vi "Milan Box.vi"() -> ()   [LabVIEW 2019]
uses:
  <vilib>/httpClient/POSTBuffer.vi
  <vilib>/httpClient/LabVIEWHTTPClient.lvlib
panel:
  out "Property (time stamp)":timestamp
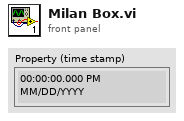
[diagram p1: front panel]
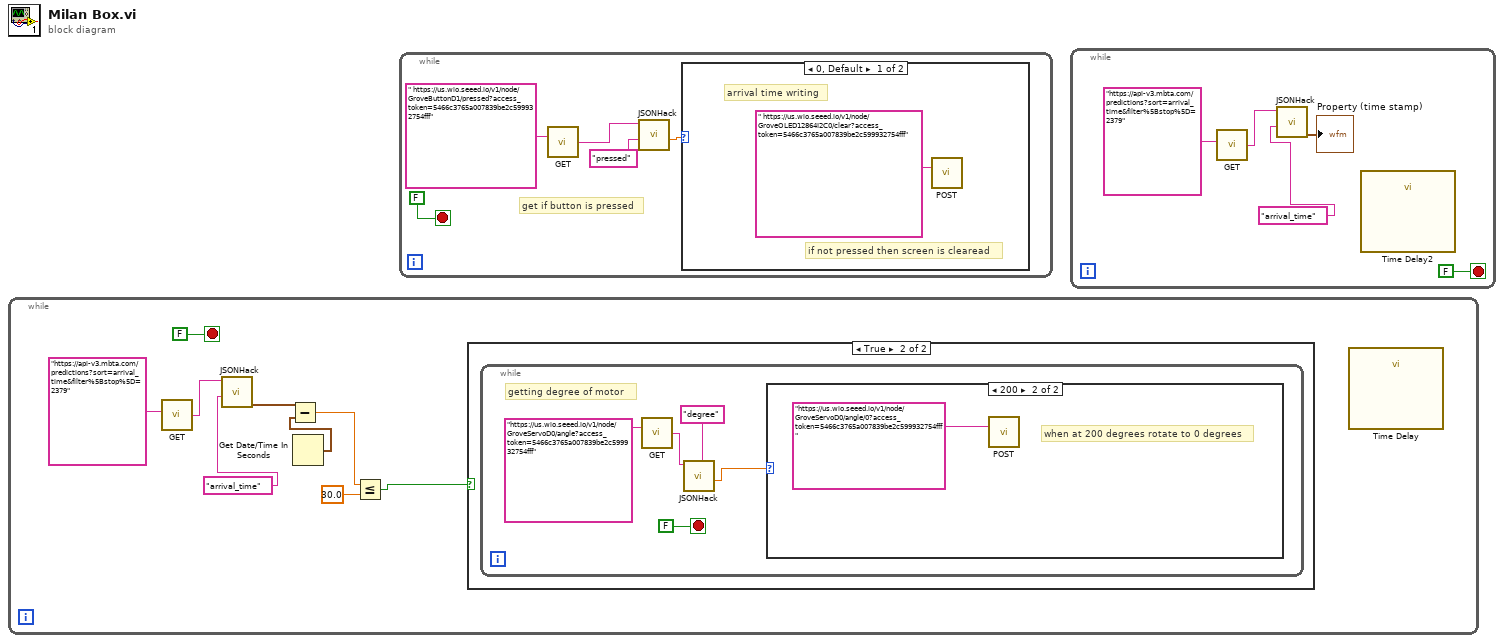
[diagram p0: block diagram]
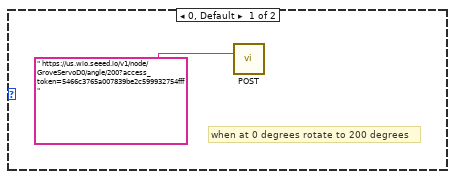
[diagram p3: hidden frame]
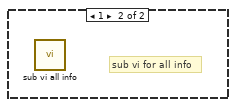
[diagram p4: hidden frame]
diagram:
  n1 = while {
    stop <- FALSE stop-if-true
    n2 = call <vilib>:"GET.vi"("url"="https://api-v3.mbta.com/predictions?sort=arrival_time&filter%5Bstop%5D=2379") -> ("body"=w8:string)  [unwired: 11 in, 3 out]
    n3 = call "JSONHack.vi"("search name"="arrival_time", "JSON in"=w8) -> ("Property (time stamp)"=w4:timestamp)  [unwired: 6 in, 3 out]
    n4 = Get Date/Time In Seconds() -> (seconds since 1Jan1904=w3:timestamp)
    n5 = Subtract(x=w4, y=w3) -> (x-y=w2:dbl)
    n6 = Less Or Equal?(x=w2, y=30.0) -> (x <= y?=w5:bool)
    n7 = case shown="True" w5 {
      frame False {
      }
      frame True {
        n8 = while {
          stop <- FALSE stop-if-true
          # "getting degree of motor"
          n9 = call <vilib>:"GET.vi"("url"="https://us.wio.seeed.io/v1/node/GroveServoD0/angle?access_token=5466c3765a007839be2c599932754fff") -> ("body"=w13:string)  [unwired: 11 in, 3 out]
          n10 = call "JSONHack.vi"("search name"="degree", "JSON in"=w13) -> ("Property (num)"=w10:dbl)  [unwired: 6 in, 3 out]
          n11 = case shown="200" w10 {
            frame 0, Default {
              # "when at 0 degrees rotate to 200 degrees"
              n12 = call-poly <vilib>:"POST.vi"("url"=" https://us.wio.seeed.io/v1/node/GroveServoD0/angle/200?access_token=5466c3765a007839be2c599932754fff") -> ()  [unwired: 11 in, 4 out]
            }
            frame 200 {
              # "when at 200 degrees rotate to 0 degrees"
              n13 = call-poly <vilib>:"POST.vi"("url"="https://us.wio.seeed.io/v1/node/GroveServoD0/angle/0?access_token=5466c3765a007839be2c599932754fff") -> ()  [unwired: 11 in, 4 out]
            }
          }
        }
      }
    }
    n14 = call "Time Delay"() -> ()  [unwired: 11 in, 1 out]
  }
  n15 = while {
    stop <- FALSE stop-if-true
    # "get if button is pressed"
    n16 = call <vilib>:"GET.vi"("url"=" https://us.wio.seeed.io/v1/node/GroveButtonD1/pressed?access_token=5466c3765a007839be2c599932754fff") -> ("body"=w20:string)  [unwired: 11 in, 3 out]
    n17 = call "JSONHack.vi"("search name"="pressed", "JSON in"=w20) -> ("Property (num)"=w19:dbl)  [unwired: 6 in, 3 out]
    n18 = case shown="0, Default" w19 {
      frame 0, Default {
        # "arrival time writing"
        # "if not pressed then screen is clearead"
        n19 = call-poly <vilib>:"POST.vi"("url"=" https://us.wio.seeed.io/v1/node/GroveOLED12864I2C0/clear?access_token=5466c3765a007839be2c599932754fff") -> ()  [unwired: 11 in, 4 out]
      }
      frame 1 {
        # "sub vi for all info"
        n20 = call "sub vi all info.vi"() -> ()  [unwired: 12 in]
      }
    }
  }
  n21 = while {
    stop <- FALSE stop-if-true
    n22 = call <vilib>:"GET.vi"("url"="https://api-v3.mbta.com/predictions?sort=arrival_time&filter%5Bstop%5D=2379") -> ("body"=w26:string)  [unwired: 11 in, 3 out]
    n23 = call "JSONHack.vi"("search name"="arrival_time", "JSON in"=w26) -> ("Property (time stamp)"=→"Property (time stamp)":timestamp)  [unwired: 6 in, 3 out]
    n24 = call "Time Delay2"() -> ()  [unwired: 11 in, 1 out]
  }
